vi "Get Data.vi"(3 "Data reg":T1 {"ЦАП, градС" format="%.3g"; "Тнагр, градС" format="%.3g"; "Q, мл" format="%.3g"; "Рдм, МПа" format="%.3g"; "Тпоп.2, мкс" format="%.3g"; "Тпоп.1, мкс" format="%.3g"; "Тпрод, мкс" format="%.3g"; "Vпл, см3" format="%.3g"; "Рэфф, МПа" format="%.3g"; "dL, мм" format="%.3g"; "R, Ом" format="%.3g"; "Ткд, градС" format="%.3g"; "Ргор, МПа" format="%.3g"; "Рпл2, МПа" format="%.3g"; "Рпл1, МПа" format="%.3g"}) -> (0 "Array of Data":string[](array[string]), 1 "Array of Headers":string[](array[string]))   [LabVIEW 2023, in "Registration.lvlib"]
uses:
  Registration.lvlib
  Data_reg.ctl
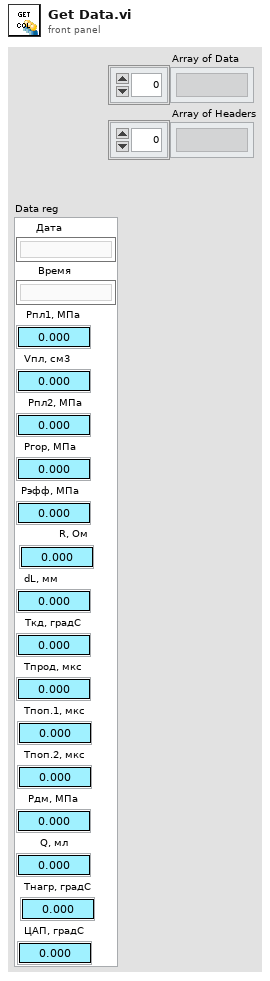
[diagram p1: front panel]
types:
  T1 = typedef "Registration.lvlib/Data_reg.ctl" = cluster{"Дата":string, "Время":string, "Рпл1, МПа":dbl, "Vпл, см3":dbl, "Рпл2, МПа":dbl, "Ргор, МПа":dbl, "Рэфф, МПа":dbl, "R, Ом":dbl, "dL, мм":dbl, "Ткд, градС":dbl, "Тпрод, мкс":dbl, "Тпоп.1, мкс":dbl, "Тпоп.2, мкс":dbl, "Рдм, МПа":dbl, "Q, мл":dbl, "Тнагр, градС":dbl, "ЦАП, градС":dbl}
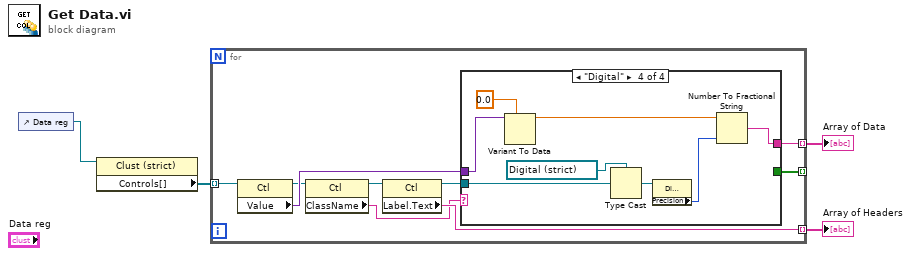
[diagram p0: block diagram]
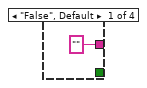
[diagram p2: hidden frame]
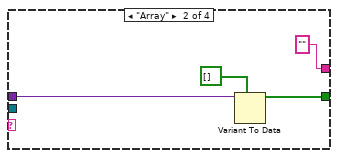
[diagram p3: hidden frame]
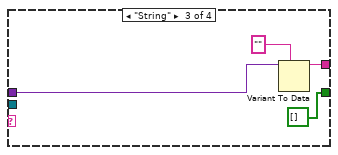
[diagram p4: hidden frame]
diagram:
  n1 = control-ref of="Data reg"() -> (w1:refnum<vi>)
  n2 = property class="Clust (strict)"(reference=w1) -> ("Controls[]"=w4:refnum<vi>[])  [unwired: 1 in, 2 out]
  n3 = for {
    tunnel: w4 -> [w13] mode=indexing
    tunnel: [w10] -> w3 mode=indexing
    tunnel: [w8] -> w2 mode=indexing
    tunnel: [w7] -> _ mode=indexing
    n4 = property class="Ctl"(reference=w13) -> (reference out=w11:refnum<vi>, "Value"=w12:variant)  [unwired: 1 in, 1 out]
    n5 = property class="Ctl"(reference=w11) -> (reference out=w9:refnum<vi>, "ClassName"=w6:string)  [unwired: 1 in, 1 out]
    n6 = property class="Ctl"(reference=w9) -> (reference out=w5:refnum<vi>, "Label.Text"=w8:string)  [unwired: 1 in, 1 out]
    n7 = case shown="\"Digital\"" w6 {
      tunnel: w12 -> [_ w17 w21 w30]
      tunnel: ["" "" w20 w27] -> w10
      tunnel: [_ w16 bool[] [] ("Array 2") _] -> w7
      tunnel: w5 -> [_ _ _ w26]
      frame "False", Default {
      }
      frame "Array" {
        n8 = Variant To Data(type=bool[] [] ("Array 2"), Variant=w17) -> (data=w16:bool[])  [unwired: 1 in, 1 out]
      }
      frame "String" {
        n9 = Variant To Data(type="", Variant=w21) -> (data=w20:string)  [unwired: 1 in, 1 out]
      }
      frame "Digital" {
        n10 = Variant To Data(type=0.0, Variant=w30) -> (data=w28:dbl)  [unwired: 1 in, 1 out]
        n11 = Type Cast(type=refnum<vi> refnum ("Numeric"), x=w26) -> (*(type *) &x=w24:refnum<vi>)
        n12 = property class="DigNum (strict)"(reference=w24) -> ("Precision"=w23:u8)  [unwired: 1 in, 2 out]
        n13 = Number To Fractional String(number=w28, precision (6)=w23) -> (F-format string=w27:string)  [unwired: 2 in]
      }
    }
  }
  "Array of Data" <- w3
  "Array of Headers" <- w2
